vi "Write Number of Steps.vi"(8 "error in (no error)":errorcluster, 10 "Number of Steps":i32=7, 11 "Frequency Measurement in":refnum<class "Frequency Measurement.lvclass">) -> (0 "error out":errorcluster, 3 "Frequency Measurement out":refnum<class "Frequency Measurement.lvclass">)   [LabVIEW 2013, in "Frequency Measurement.lvlib" / "Frequency Measurement.lvclass"]
uses:
  Frequency Measurement.lvclass
  Frequency Measurement.lvclass/Frequency Measurement.ctl
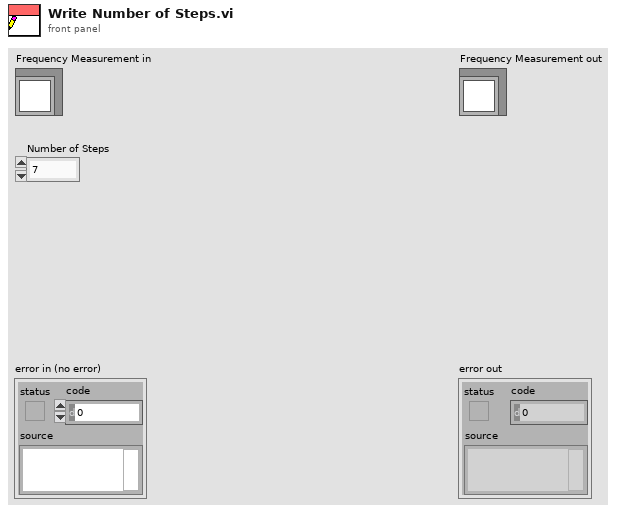
[diagram p1: front panel]
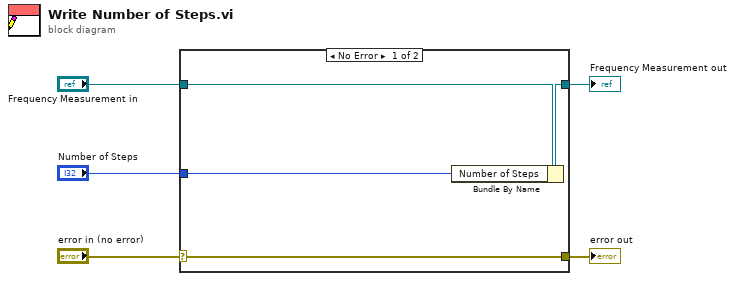
[diagram p0: block diagram]
diagram:
  n1 = case shown="No Error" "error in (no error)" {
    selector: "error in (no error)" -> [w9 w10]
    tunnel: [w9 w10] -> w4
    tunnel: [w7 w11] -> w2
    tunnel: "Frequency Measurement in" -> [w8 w11]
    tunnel: "Number of Steps" -> [w6 _]
    frame No Error {
      n2 = Bundle By Name(cluster=w8, "Number of Steps"=w6) -> (w7:refnum<class "Frequency Measurement.lvclass">)
    }
    frame Error {
    }
  }
  "error out" <- w4
  "Frequency Measurement out" <- w2
